vi "listbox_drag_drop.vi"() -> ()   [LabVIEW 2021]
panel:
  in  "stop":bool
  in  "Listbox 2":i32(listbox)=2
  in  "Listbox":i32(listbox)
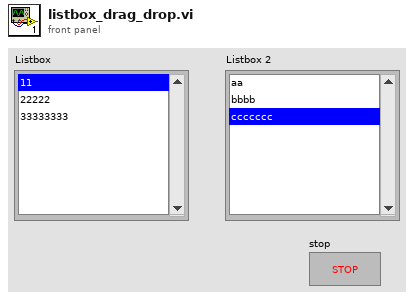
[diagram p1: front panel]
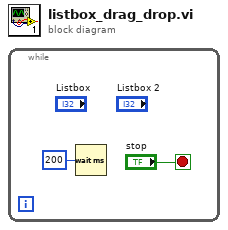
[diagram p0: block diagram]
diagram:
  n1 = while {
    stop <- "stop" stop-if-true
    n2 = Wait (ms)(milliseconds to wait=u32 200) -> ()  [unwired: 1 out]
  }
